vi "Create path.vi"(8 "error in (no error)":errorcluster, 11 "Retiga in":refnum<class "Retiga.lvclass">) -> (0 "error out":errorcluster, 2 "full path":path, 3 "Retiga out":refnum<class "Retiga.lvclass">)   [LabVIEW 2012, in "Retiga.lvclass"]
uses:
  Retiga.lvclass
  Retiga.lvclass/Retiga.ctl
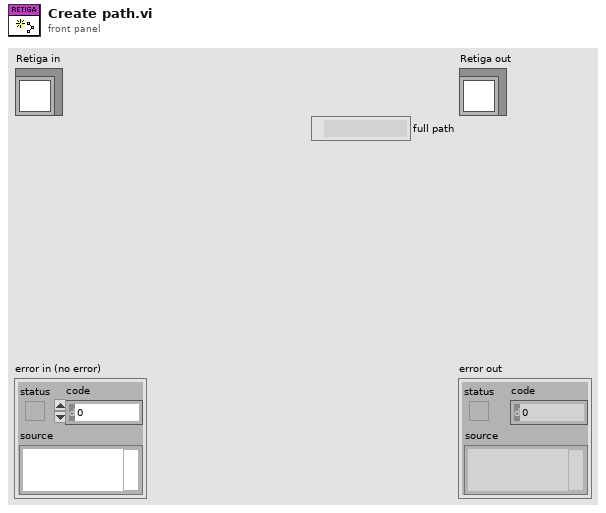
[diagram p1: front panel]
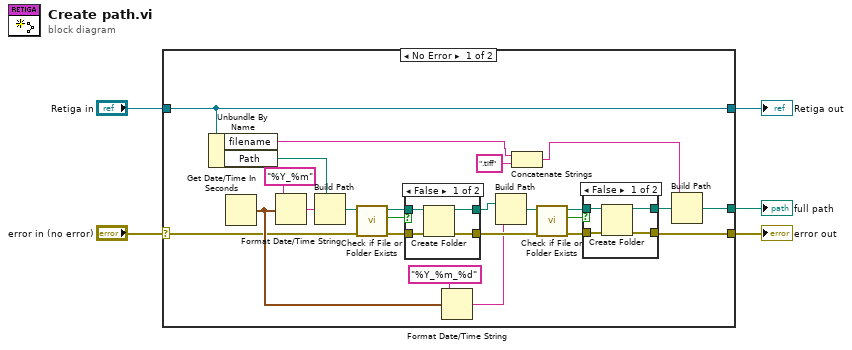
[diagram p0: block diagram]
diagram:
  n1 = case shown="No Error" "error in (no error)" {
    selector: "error in (no error)" -> [w8 w43]
    tunnel: [w7 w43] -> w4
    tunnel: [w9 w42] -> w2
    tunnel: "Retiga in" -> [w9 w42]
    tunnel: [w6 _] -> w1
    frame No Error {
      n2 = Unbundle By Name(w9) -> ("filename"=w11:string, "Path"=w26:path)
      n3 = Get Date/Time In Seconds() -> (seconds since 1Jan1904=w17:timestamp)
      n4 = Format Date/Time String(time format string (%c)="%Y_%m", seconds (now)=w17) -> (date/time string=w28:string)  [unwired: 1 in]
      n5 = Build Path(base path=w26, name or relative path=w28) -> (appended path=w29:path)
      n6 = call <vilib>:"Check if File or Folder Exists.vi"("error in (no error)"=w8, "path"=w29) -> ("error out"=w20:errorcluster, "file or folder exists?"=w18:bool, "dup path"=w19:path)  [unwired: 7 in]
      n7 = case shown="False" w18 {
        tunnel: w20 -> [w39 w41]
        tunnel: w19 -> [w38 w40]
        tunnel: [w37 w41] -> w24
        tunnel: [w36 w40] -> w25
        frame False {
          n8 = Create Folder(path (use dialog)=w38, error in=w39) -> (created path=w36:path, error out=w37:errorcluster)  [unwired: 1 in, 1 out]
        }
        frame True {
        }
      }
      n9 = Format Date/Time String(time format string (%c)="%Y_%m_%d", seconds (now)=w17) -> (date/time string=w22:string)  [unwired: 1 in]
      n10 = Build Path(base path=w25, name or relative path=w22) -> (appended path=w21:path)
      n11 = Concatenate Strings(w11, ".tiff" ("string")) -> (w10:string)
      n12 = call <vilib>:"Check if File or Folder Exists.vi"("error in (no error)"=w24, "path"=w21) -> ("error out"=w15:errorcluster, "file or folder exists?"=w14:bool, "dup path"=w16:path)  [unwired: 7 in]
      n13 = case shown="False" w14 {
        tunnel: w15 -> [w33 w35]
        tunnel: w16 -> [w32 w34]
        tunnel: [w31 w35] -> w7
        tunnel: [w30 w34] -> w13
        frame False {
          n14 = Create Folder(path (use dialog)=w32, error in=w33) -> (created path=w30:path, error out=w31:errorcluster)  [unwired: 1 in, 1 out]
        }
        frame True {
        }
      }
      n15 = Build Path(base path=w13, name or relative path=w10) -> (appended path=w6:path)
    }
    frame Error {
    }
  }
  "error out" <- w4
  "Retiga out" <- w2
  "full path" <- w1
